vi "get enum.vi"(8 "error in (no error)":errorcluster, 11 "path":string) -> (0 "error out":errorcluster, 3 "Enum Elements":string[](array[string]))   [LabVIEW 2020]
doc: "Returns the elements of an enum stored in a .ctl file specified by path. Use this to see which elements a type-defined enum has."
uses:
  G-AI Core/G-AI Core.lvlib
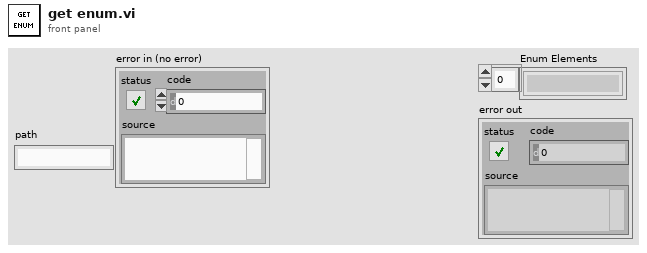
[diagram p1: front panel]
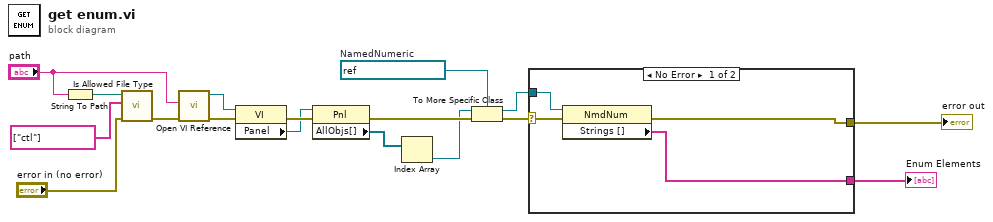
[diagram p0: block diagram]
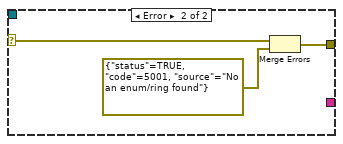
[diagram p2: hidden frame]
diagram:
  w9 = refnum<vi> refnum  # NamedNumeric
  n1 = String To Path(string="path") -> (path=w5:path)
  n2 = call "Is Allowed File Type.vi"("error in (no error)"="error in (no error)", "y"=string[] ["ctl"], "Path"=w5) -> ("error out"=w4:errorcluster)  [unwired: 8 in]
  n3 = call "Open VI Reference.vi"("error in"=w4, "VI Path"="path") -> ("error out"=w17:errorcluster, "VI Refnum"=w16:refnum<vi>)  [unwired: 8 in]
  n4 = property class="VI"(reference=w16, error in=w17) -> (error out=w15:errorcluster, "Panel"=w14:refnum<vi>)  [unwired: 1 out]
  n5 = property class="Pnl"(reference=w14, error in=w15) -> (error out=w12:errorcluster, "AllObjs[]"=w13:refnum<vi>[])  [unwired: 1 out]
  n6 = Index Array(array=w13) -> (element=w11:refnum<vi>)  [unwired: 1 in]
  n7 = To More Specific Class(target class=w9, reference=w11, error in=w12) -> (specific class reference=w10:refnum<vi>, error out=w6:errorcluster)
  n8 = case shown="No Error" w6 {
    selector: w6 -> [w18 w22]
    tunnel: w10 -> [w21 _]
    tunnel: [w20 _] -> w8
    tunnel: [w19 w23] -> w7
    frame No Error {
      n9 = property class="NmdNum"(reference=w21, error in=w18) -> (error out=w19:errorcluster, "Strings []"=w20:string[])  [unwired: 1 out]
    }
    frame Error {
      n10 = Merge Errors(w22, errorcluster {"status"=TRUE, "code"=5001, "source"="No an enum/ring found"} ("error out")) -> (w23:errorcluster)
    }
  }
  "Enum Elements" <- w8
  "error out" <- w7
